vi "KE2400_Set_Volt_Meas_Current.vi"(4 "Manual Settling Delay (0 sec)":dbl, 6 "Enable Auto Range (T:Enable)":bool=TRUE, 7 "Compliance  Level (0.1)":dbl=0.1, 8 "error in (no error)":errorcluster, 9 "Enable Remote Sensing (T: Enable)":bool=TRUE, 10 "Output Level (0)":dbl, 11 "VISA resource name":refnum<visa-resource-name>) -> (0 "error out":errorcluster, 1 "Current":sgl, 2 "Voltage":sgl)   [LabVIEW 2017]
uses:
  Instrument Drivers/keithley_24xx/Keithley 24XX/Public/Data/Read (Single Point).vi
  Instrument Drivers/keithley_24xx/Keithley 24XX/Keithley 24XX.lvlib
panel:
  in  "Manual Range (1.0)":dbl=100.0 format="%#_13g"
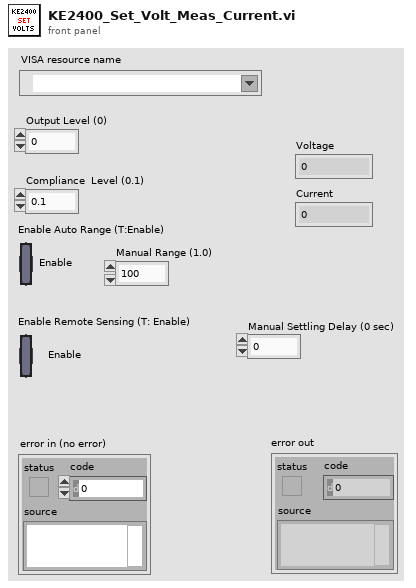
[diagram p1: front panel]
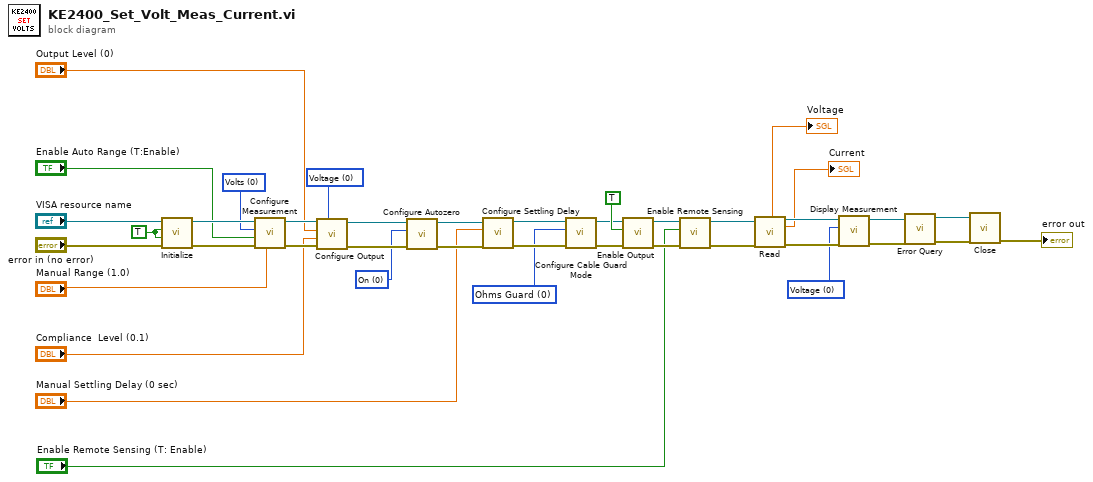
[diagram p0: block diagram]
diagram:
  w7 = u16 0 items=["Voltage", "Current", "Resistance"] ("Displayed Measurement (0: Voltage)")
  w19 = u16 0 items=["Ohms Guard", "Cable Guard"] ("Guard Mode  (0: Ohms Guard)")
  w25 = u16 0 items=["On", "Off", "Once"] ("Autozero  (0: On)")
  w28 = TRUE ("ID Query (True)")
  w32 = u16 0 items=["Volts", "Current", "Resistance"] ("Function (0: Volts)")
  w34 = u16 0 items=["Voltage", "Current"] ("Source Mode  (0: Voltage)")
  n1 = call "Initialize.vi"("error in (no error)"="error in (no error)", "Reset (True)"=w28, "ID Query (True)"=w28, "VISA resource name"="VISA resource name") -> ("error out"=w40:errorcluster, "VISA resource name out"=w39:refnum<visa-resource-name>)  [unwired: 6 in]
  n2 = call "Configure Measurement.vi"("Manual Range (1.0)"="Manual Range (1.0)", "error in (no error)"=w40, "Enable Auto Range (T:Enable)"="Enable Auto Range (T:Enable)", "Function (0: Volts)"=w32, "VISA resource name"=w39) -> ("error out"=w37:errorcluster, "VISA resource name out"=w38:refnum<visa-resource-name>)  [unwired: 5 in]
  n3 = call "Configure Output.vi"("Source Mode  (0: Voltage)"=w34, "error in (no error)"=w37, "Compliance  Level (0.1)"="Compliance  Level (0.1)", "Output Level (0)"="Output Level (0)", "VISA resource name"=w38) -> ("error out"=w27:errorcluster, "VISA resource name out"=w26:refnum<visa-resource-name>)  [unwired: 5 in]
  n4 = call "Configure Autozero.vi"("error in (no error)"=w27, "Autozero  (0: On)"=w25, "VISA resource name"=w26) -> ("error out"=w24:errorcluster, "VISA resource name out"=w23:refnum<visa-resource-name>)  [unwired: 7 in]
  n5 = call "Configure Settling Delay.vi"("error in (no error)"=w24, "Manual Settling Delay (0 sec)"="Manual Settling Delay (0 sec)", "VISA resource name"=w23) -> ("error out"=w21:errorcluster, "VISA resource name out"=w20:refnum<visa-resource-name>)  [unwired: 7 in]
  n6 = call "Configure Cable Guard Mode.vi"("error in (no error)"=w21, "Guard Mode  (0: Ohms Guard)"=w19, "VISA resource name"=w20) -> ("error out"=w16:errorcluster, "VISA resource name out"=w17:refnum<visa-resource-name>)  [unwired: 7 in]
  n7 = call "Enable Output.vi"("error in (no error)"=w16, "Enable Output (T: Enable)"=TRUE, "VISA resource name"=w17) -> ("error out"=w15:errorcluster, "VISA resource name out"=w14:refnum<visa-resource-name>)  [unwired: 7 in]
  n8 = call "Enable Remote Sensing.vi"("error in (no error)"=w15, "Enable Remote Sensing (T: Enable)"="Enable Remote Sensing (T: Enable)", "VISA resource name"=w14) -> ("error out"=w12:errorcluster, "VISA resource name out"=w11:refnum<visa-resource-name>)  [unwired: 7 in]
  n9 = call-poly "Read.vi"("VISA resource name"=w11, "error in (no error)"=w12) -> ("Voltage"=→"Voltage":sgl, "VISA resource name out"=w9:refnum<visa-resource-name>, "Current"=→"Current":sgl, "error out"=w10:errorcluster)  [unwired: 7 in, 3 out]
  n10 = call "Display Measurement.vi"("error in (no error)"=w10, "Displayed Measurement (0: Voltage)"=w7, "VISA resource name"=w9) -> ("error out"=w5:errorcluster, "VISA resource name out"=w4:refnum<visa-resource-name>)  [unwired: 7 in]
  n11 = call "Error Query.vi"("error in (no error)"=w5, "VISA resource name"=w4) -> ("error out"=w3:errorcluster, "VISA resource name out"=w2:refnum<visa-resource-name>)  [unwired: 6 in, 2 out]
  n12 = call "Close.vi"("error in (no error)"=w3, "VISA resource name"=w2) -> ("error out"=→"error out":errorcluster)  [unwired: 9 in]
